vi "WAV_parse.vi"(11 "Chunks":T1(array[cluster])) -> (0 "Parameters":string[][](table), 1 "Graph":waveform(dbl)[](graph), 3 "format":T2)   [LabVIEW 2022 SP3]
uses:
  <vilib>/Utility/error.llb/Trim Whitespace One-Sided.vi
panel:
  out "info":T1(array[cluster])
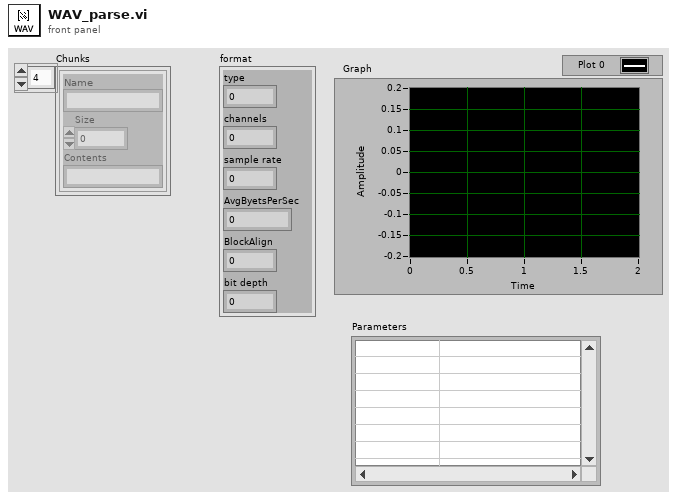
[diagram p1: front panel]
types:
  T1 = cluster{"Name":string, "Size":u32, "Contents":string}[]
  T2 = cluster{"type":u16, "channels":u16, "sample rate":u32, "AvgByetsPerSec":u32, "BlockAlign":u16, "bit depth":u16}
  T3 = enum16{"big-endian, network order", "native, host order", "little-endian"}
  T4 = cluster{"u16":u16, "u16":u16, "u32":u32, "u32":u32, "u16":u16, "u16":u16}
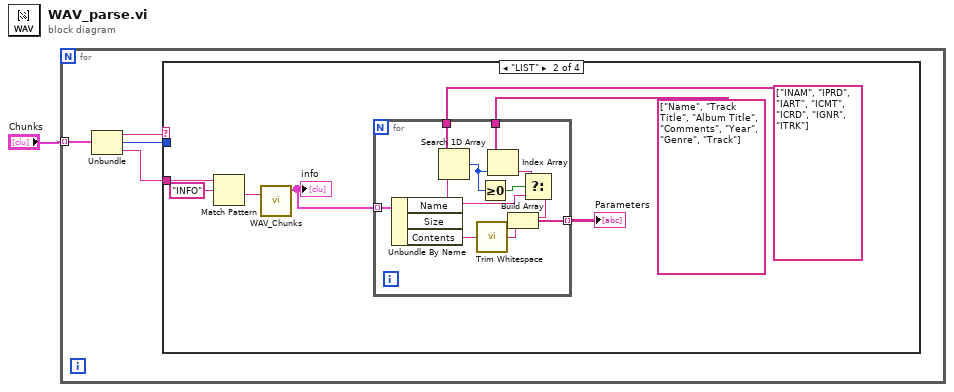
[diagram p0: block diagram]
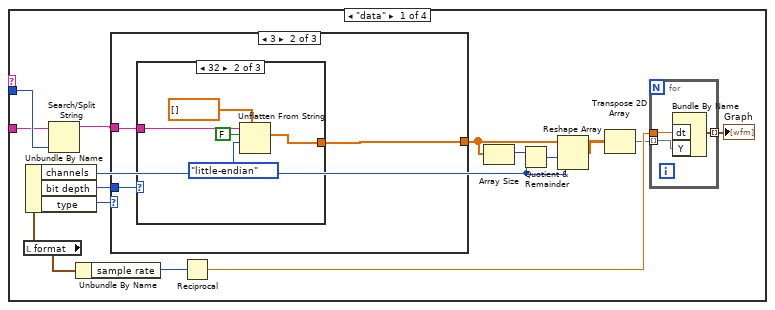
[diagram p2: hidden frame]
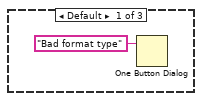
[diagram p3: hidden frame]
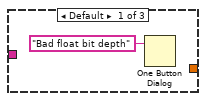
[diagram p4: hidden frame]
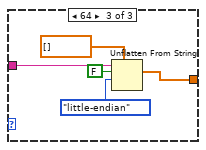
[diagram p5: hidden frame]
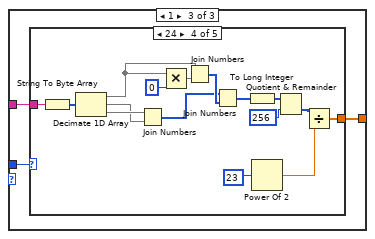
[diagram p6: hidden frame]
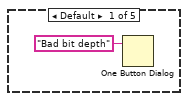
[diagram p7: hidden frame]
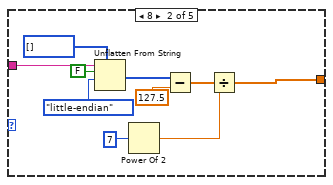
[diagram p8: hidden frame]
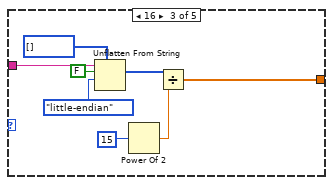
[diagram p9: hidden frame]
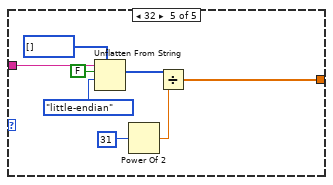
[diagram p10: hidden frame]
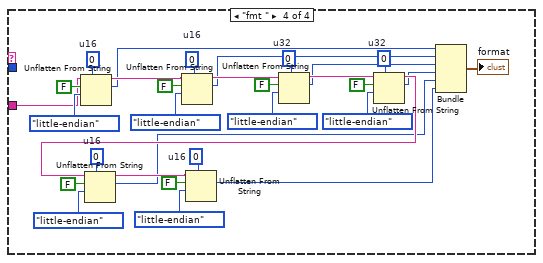
[diagram p12: hidden frame]
diagram:
  n1 = for {
    tunnel: "Chunks" -> [w5] mode=indexing
    n2 = Unbundle(w5) -> ("Name"=w4:string, "Size"=w3:u32, "Contents"=w2:string)
    n3 = case shown="\"LIST\"" w4 {
      tunnel: w2 -> [w12 w91 _ w130]
      tunnel: w3 -> [w18 _ _ _]
      frame "data" {
        n4 = local read "format"() -> (w16:T2)
        n5 = Unbundle By Name(w16) -> ("channels"=w7:u16, "bit depth"=w19:u16, "type"=w20:u16)
        n6 = Search/Split String(string=w12, offset (0)=w18) -> (substring before match=w17:string)  [unwired: 1 in, 2 out]
        n7 = Unbundle By Name(w16) -> ("sample rate"=w15:u32)
        n8 = case shown="3" w20 {
          tunnel: w19 -> [_ w26 w40]
          tunnel: w17 -> [_ w27 w41]
          tunnel: [_ w25 w39] -> w10
          frame Default {
            n9 = One Button Dialog(message="Bad format type") -> ()  [unwired: 1 in, 1 out]
          }
          frame 3 {
            n10 = case shown="32" w26 {
              tunnel: w27 -> [_ w31 w35]
              tunnel: [_ w30 w34] -> w25
              frame Default {
                n11 = One Button Dialog(message="Bad float bit depth") -> ()  [unwired: 1 in, 1 out]
              }
              frame 32 {
                n12 = Unflatten From String(type=sgl[] [], binary string=w31, data includes array or string size? (T)=FALSE, byte order (0:big-endian, network order)=T3."little-endian") -> (value=w30:sgl[])  [unwired: 1 in, 2 out]
              }
              frame 64 {
                n13 = Unflatten From String(type=dbl[] [], binary string=w35, data includes array or string size? (T)=FALSE, byte order (0:big-endian, network order)=T3."little-endian") -> (value=w34:dbl[])  [unwired: 1 in, 2 out]
              }
            }
          }
          frame 1 {
            n14 = case shown="24" w40 {
              tunnel: w41 -> [_ w50 w59 w62 w82]
              tunnel: [_ w45 w56 w76 w79] -> w39
              frame Default {
                n15 = One Button Dialog(message="Bad bit depth") -> ()  [unwired: 1 in, 1 out]
              }
              frame 8 {
                n16 = Unflatten From String(type=u8[] [], binary string=w50, data includes array or string size? (T)=FALSE, byte order (0:big-endian, network order)=T3."little-endian") -> (value=w44:u8[])  [unwired: 1 in, 2 out]
                n17 = Power Of 2(x=7 ("count")) -> (2^x=w47:dbl)
                n18 = Subtract(x=w44, y=127.5 ("count")) -> (x-y=w43:dbl[])
                n19 = Divide(x=w43, y=w47) -> (x/y=w45:dbl[])
              }
              frame 16 {
                n20 = Unflatten From String(type=i16[] [], binary string=w59, data includes array or string size? (T)=FALSE, byte order (0:big-endian, network order)=T3."little-endian") -> (value=w57:i16[])  [unwired: 1 in, 2 out]
                n21 = Power Of 2(x=15 ("count")) -> (2^x=w54:dbl)
                n22 = Divide(x=w57, y=w54) -> (x/y=w56:dbl[])
              }
              frame 24 {
                n23 = String To Byte Array(string=w62) -> (unsigned byte array=w65:u8[])
                n24 = Decimate 1D Array(w65) -> (w66:u8[], w70:u8[], w71:u8[])
                n25 = Join Numbers(hi=w71, lo=w70) -> ((hi.lo)=w69:u16[])
                n26 = Multiply(x=w66, y=u8 0) -> (x*y=w67:u8[])
                n27 = Join Numbers(hi=w66, lo=w67) -> ((hi.lo)=w73:u16[])
                n28 = Join Numbers(hi=w69, lo=w73) -> ((hi.lo)=w72:u32[])
                n29 = To Long Integer(number=w72) -> (32bit integer=w68:i32[])
                n30 = Power Of 2(x=23 ("count")) -> (2^x=w74:dbl)
                n31 = Quotient & Remainder(x=w68, y=256) -> (floor(x/y)=w61:i32[])  [unwired: 1 out]
                n32 = Divide(x=w61, y=w74) -> (x/y=w76:dbl[])
              }
              frame 32 {
                n33 = Unflatten From String(type=i32[] [], binary string=w82, data includes array or string size? (T)=FALSE, byte order (0:big-endian, network order)=T3."little-endian") -> (value=w80:i32[])  [unwired: 1 in, 2 out]
                n34 = Power Of 2(x=31 ("count")) -> (2^x=w77:dbl)
                n35 = Divide(x=w80, y=w77) -> (x/y=w79:dbl[])
              }
            }
          }
        }
        n36 = Reciprocal(x=w15) -> (1/x=w14:dbl)
        n37 = Array Size(array=w10) -> (size(s)=w9:i32)
        n38 = Quotient & Remainder(x=w9, y=w7) -> (floor(x/y)=w8:i32)  [unwired: 1 out]
        n39 = Reshape Array(w10, w8, w7) -> (w11:dbl[][])
        n40 = Transpose 2D Array(2D array=w11) -> (transposed array=w6:dbl[][])
        n41 = for {
          tunnel: w14 -> [w23]
          tunnel: w6 -> [w22] mode=indexing
          tunnel: [w21] -> w13 mode=indexing
          n42 = Bundle By Name("dt"=w23, "Y"=w22) -> (w21:waveform(dbl))  [unwired: 1 in]
        }
        "Graph" <- w13
      }
      frame "LIST" {
        n43 = Match Pattern(string=w91, regular expression="INFO") -> (after substring=w89:string)  [unwired: 1 in, 3 out]
        n44 = call "WAV_Chunks.vi"("contents"=w89) -> ("Chunks"=w88:T1)  [unwired: 10 in]
        "info" <- w88
        n45 = for {
          tunnel: w88 -> [w102] mode=indexing
          tunnel: [w99] -> w87 mode=indexing
          tunnel: string[] ["INAM", "IPRD", "IART", "ICMT", "ICRD", "IGNR", "ITRK"] -> [w98]
          tunnel: string[] ["Name", "Track Title", "Album Title", "Comments", "Year", "Genre", "Track"] -> [w97]
          n46 = Unbundle By Name(w102) -> ("Name"=w93:string, "Contents"=w101:string)  [unwired: 1 out]
          n47 = Search 1D Array(1D array=w98, element=w93) -> (index of element=w96:i32)  [unwired: 1 in]
          n48 = call <vilib>:"Trim Whitespace.vi"("string"=w101) -> ("trimmed string"=w100:string)  [unwired: 1 in]
          n49 = Greater Or Equal To 0?(x=w96) -> (x >= 0?=w95:bool)
          n50 = Index Array(array=w97, index=w96) -> (element=w94:string)
          n51 = Select(t=w94, s=w95, f=w93) -> (s? t:f=w92:string)
          n52 = Build Array(w92, w100) -> (w99:string[])
        }
        "Parameters" <- w87
      }
      frame Default {
      }
      frame "fmt " {
        w118 = u16 0  # u16
        w113 = u16 0  # u16
        w106 = u32 0  # u32
        w125 = u32 0  # u32
        w126 = u16 0  # u16
        w132 = u16 0  # u16
        n53 = Unflatten From String(type=w132, binary string=w130, data includes array or string size? (T)=FALSE, byte order (0:big-endian, network order)=T3."little-endian") -> (rest of the binary string=w127:string, value=w110:u16)  [unwired: 1 in, 1 out]
        n54 = Unflatten From String(type=w126, binary string=w127, data includes array or string size? (T)=FALSE, byte order (0:big-endian, network order)=T3."little-endian") -> (rest of the binary string=w122:string, value=w109:u16)  [unwired: 1 in, 1 out]
        n55 = Unflatten From String(type=w125, binary string=w122, data includes array or string size? (T)=FALSE, byte order (0:big-endian, network order)=T3."little-endian") -> (rest of the binary string=w119:string, value=w108:u32)  [unwired: 1 in, 1 out]
        n56 = Unflatten From String(type=w106, binary string=w119, data includes array or string size? (T)=FALSE, byte order (0:big-endian, network order)=T3."little-endian") -> (rest of the binary string=w111:string, value=w107:u32)  [unwired: 1 in, 1 out]
        n57 = Unflatten From String(type=w113, binary string=w111, data includes array or string size? (T)=FALSE, byte order (0:big-endian, network order)=T3."little-endian") -> (rest of the binary string=w117:string, value=w105:u16)  [unwired: 1 in, 1 out]
        n58 = Unflatten From String(type=w118, binary string=w117, data includes array or string size? (T)=FALSE, byte order (0:big-endian, network order)=T3."little-endian") -> (value=w104:u16)  [unwired: 1 in, 2 out]
        n59 = Bundle("u16"=w110, "u16"=w109, "u32"=w108, "u32"=w107, "u16"=w105, "u16"=w104) -> (→"format":T4)  [unwired: 1 in]
      }
    }
  }
